vi "Scale Freq Data.vi"(0 "Data Read":dbl[](array[numeric]), 12 "Signal Coefficients":cluster{"Coefficients":dbl[]}={"Coefficients"=[1.0]}) -> (4 "Scaled Data":dbl[](array[numeric]))   [LabVIEW 2019]
uses:
  <vilib>/Analysis/NI_AALBase.lvlib
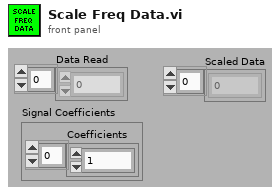
[diagram p1: front panel]
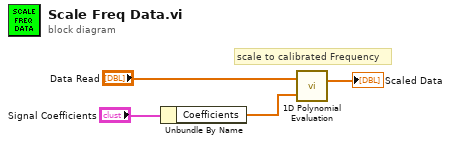
[diagram p0: block diagram]
diagram:
  # "scale to calibrated Frequency"
  n1 = Unbundle By Name("Signal Coefficients") -> ("Coefficients"=w4:dbl[])
  n2 = call <vilib>:"1D Polynomial Evaluation.vi"("Coefficients: a"=w4, "X"="Data Read") -> ("Y"=→"Scaled Data":dbl[])  [unwired: 1 out]
